vi "settings.vi"(3 "values":dbl[](array[numeric]), 5 "sturing in":refnum<visa-resource-name>) -> (1 "sturing out":refnum<visa-resource-name>)   [LabVIEW 2018]
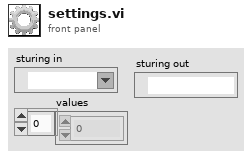
[diagram p1: front panel]
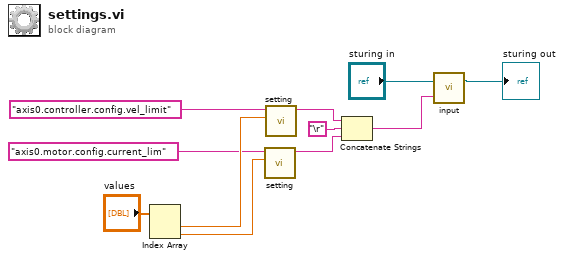
[diagram p0: block diagram]
diagram:
  n1 = Index Array(array="values") -> (element #1=w10:dbl, element #2=w6:dbl)  [unwired: 2 in]
  n2 = call "setting.vi"("value"=w6, "setting"="axis0.motor.config.current_lim") -> ("write"=w4:string)  [unwired: 9 in]
  n3 = call "setting.vi"("value"=w10, "setting"="axis0.controller.config.vel_limit") -> ("write"=w8:string)  [unwired: 9 in]
  n4 = Concatenate Strings(w8, "\r", w4) -> (w9:string)
  n5 = call "input.vi"("commando"=w9, "VISA in"="sturing in") -> ("VISA out"=→"sturing out":refnum<visa-resource-name>)  [unwired: 1 out]
